vi "SFC_Daught Board Process Check.vi"(6 "UserNo":string, 7 "ChildSN":string, 8 "error in (no error)":errorcluster caption="错误输入（无错误）", 9 "ParentSN":string, 10 "Process":string, 11 "Traceability 引用句柄":refnum<k24>) -> (0 "error out":errorcluster caption="错误输出", 2 "SFC_DaughtBoardProcessCheck":string, 3 "Traceability 引用句柄输出":refnum<k24>)   [LabVIEW 2014, in "Traceability.lvlib"]
uses:
  D:/webservice/Traceability.dll
  Traceability.dll
  Traceability.lvlib
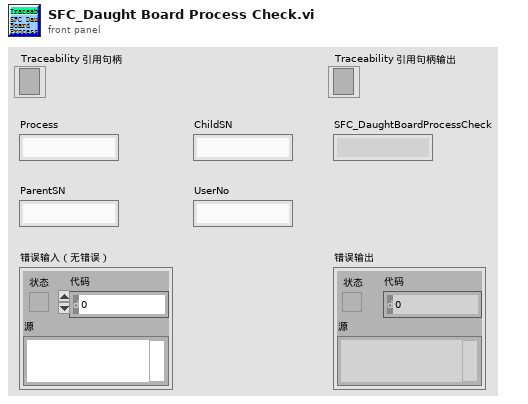
[diagram p1: front panel]
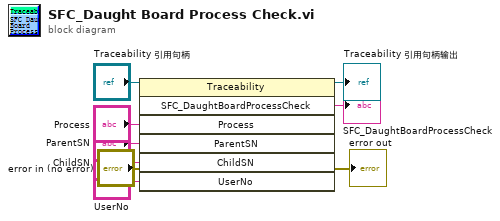
[diagram p0: block diagram]
diagram:
  n1 = invoke class="Traceability" method="SFC_DaughtBoardProcessCheck"(reference="Traceability 引用句柄", error in="error in (no error)", "Process"="Process", "ParentSN"="ParentSN", "ChildSN"="ChildSN", "UserNo"="UserNo") -> (reference out=→"Traceability 引用句柄输出":refnum<k24>, error out=→"error out":errorcluster, "SFC_DaughtBoardProcessCheck"=→"SFC_DaughtBoardProcessCheck":string)  [unwired: 1 in, 4 out]
